vi "Trigger Limit Reached.vi"(4 "Timeout Limit Reached":bool, 6 "Character Count Limit Reached":bool, 7 "Full String":string, 9 "Response In":string, 10 "Remaining string in":string) -> (1 "Response out":string, 2 "Remaining string out":string)   [LabVIEW 2017, in "SSH.lvlib"]
doc: "If the Timeout Limit or Character Count Limit has been reached, output the entire buffer string and set the remaining string to be empty"
uses:
  SSH.lvlib
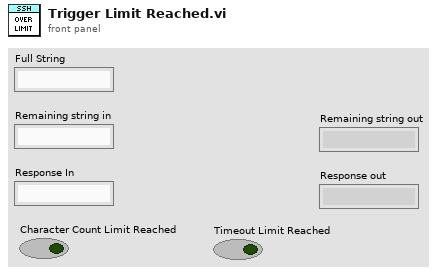
[diagram p1: front panel]
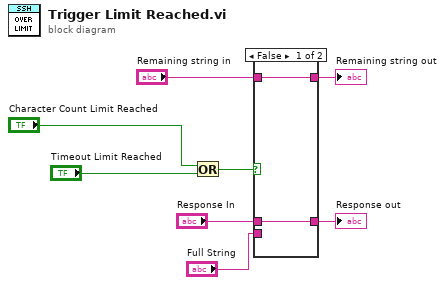
[diagram p0: block diagram]
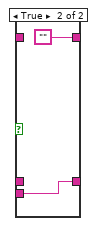
[diagram p2: hidden frame]
diagram:
  n1 = Or(x="Character Count Limit Reached", y="Timeout Limit Reached") -> (x .or. y?=w1:bool)
  n2 = case shown="False" w1 {
    tunnel: "Remaining string in" -> [w10 _]
    tunnel: [w10 ""] -> w5
    tunnel: [w9 w12] -> w6
    tunnel: "Response In" -> [w9 _]
    tunnel: "Full String" -> [_ w12]
    frame False {
    }
    frame True {
    }
  }
  "Response out" <- w6
  "Remaining string out" <- w5
